vi "Configure Limit Test Null Offset.vi"(5 "Auto Null Offset  (F: Disable)":bool, 6 "Limit Test Null Offset (0)":dbl, 7 "Enable Limit Test Null Offset (F: Disable)":bool, 8 "error in (no error)":errorcluster, 10 "Channel (0: Channel 1)":i32(ring) items=["Channel 1", "Channel 2"], 11 "VISA resource name":refnum<visa-resource-name>) -> (0 "error out":errorcluster, 3 "VISA resource name out":refnum<visa-resource-name>)   [LabVIEW 2020, in "Agilent B2900 Series.lvlib"]
doc: "Change the settings for the null offset function for cancelling the offset value from the measurement data automatically.\n\n<B>Note:</B>\nThis VI is not applicable for Agilent models B2961A, B2962A, B2961B and B2962B"
uses:
  Agilent B2900 Series.lvlib
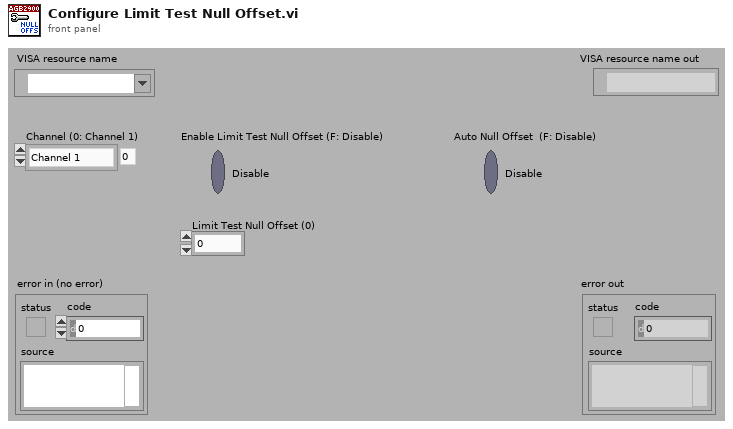
[diagram p1: front panel]
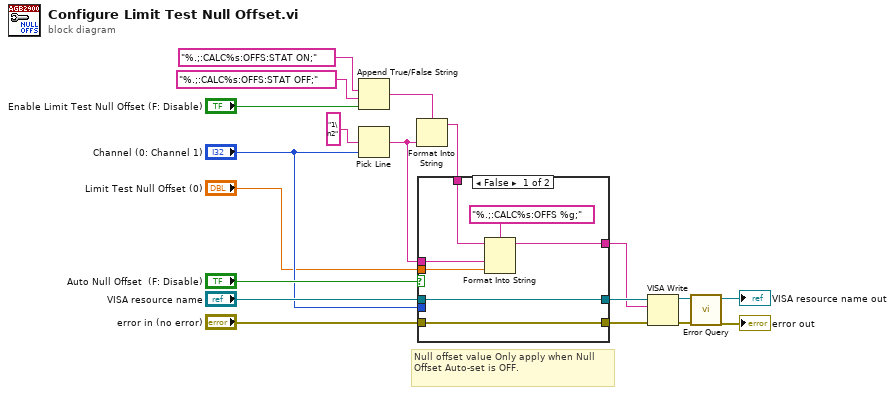
[diagram p0: block diagram]
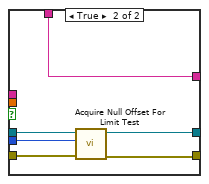
[diagram p2: hidden frame]
diagram:
  # "Null offset value Only apply when Null Offset Auto-set is OFF."
  n1 = Append True/False String(1:"Enable Limit Test Null Offset (F: Disable)", 2:"%.;:CALC%s:OFFS:STAT OFF;", 3:"%.;:CALC%s:OFFS:STAT ON;") -> (0:w7:string)  [unwired: 1 in]
  n2 = Pick Line(multi-line string="1\n2" ("string (\"\")"), line index="Channel (0: Channel 1)") -> (output string=w1:string)  [unwired: 1 in]
  n3 = Format Into String(format string=w7, w1) -> (resulting string=w2:string)  [unwired: 2 in, 1 out]
  n4 = case shown="False" "Auto Null Offset  (F: Disable)" {
    tunnel: "Channel (0: Channel 1)" -> [_ w32]
    tunnel: "VISA resource name" -> [w26 w31]
    tunnel: "error in (no error)" -> [w25 w30]
    tunnel: [w26 w29] -> w10
    tunnel: [w25 w28] -> w9
    tunnel: w2 -> [w21 w27]
    tunnel: "Limit Test Null Offset (0)" -> [w24 _]
    tunnel: [w23 w27] -> w3
    tunnel: w1 -> [w20 _]
    frame False {
      n5 = Format Into String(format string="%.;:CALC%s:OFFS %g;", initial string=w21, w20, w24) -> (resulting string=w23:string)  [unwired: 1 in, 1 out]
    }
    frame True {
      n6 = call "Acquire Null Offset For Limit Test.vi"("error in (no error)"=w30, "Channel (0: Channel 1)"=w32, "VISA resource name"=w31) -> ("error out"=w28:errorcluster, "VISA resource name out"=w29:refnum<visa-resource-name>)  [unwired: 6 in, 1 out]
    }
  }
  n7 = VISA Write(VISA resource name=w10, write buffer=w3, error in (no error)=w9) -> (VISA resource name out=w16:refnum<visa-resource-name>, error out=w15:errorcluster)  [unwired: 1 out]
  n8 = call "Error Query.vi"("error in (no error)"=w15, "VISA resource name"=w16) -> ("error out"=→"error out":errorcluster, "VISA resource name out"=→"VISA resource name out":refnum<visa-resource-name>)  [unwired: 6 in, 2 out]
